vi "Initialize.vi"(8 "error in (no error)":errorcluster, 11 "Modbus master in":refnum<class "Modbus Master.lvclass">) -> (0 "error out":errorcluster, 3 "Modbus master out":refnum<class "Modbus Master.lvclass">)   [LabVIEW 2021, in "Modbus Master.lvclass"]
doc: "Initializes a Modbus master instance. If using the <B>Create Modbus Instance</B> VI, this is not necessary. This function will initiate any required bus communication."
uses:
  Modbus Master.lvclass
  D:/my_projects/projects/Algorithms/Labview/21/Modbus_v121c/API/Modbus API.lvclass
  Modbus API.lvclass/Modbus API.ctl
  Read Network Protocol.vi
  Network Protocol/Network Master/Network Master.lvclass
  D:/my_projects/projects/Algorithms/Labview/21/Modbus_v121c/Network Protocol/Network Protocol.lvclass
  Modbus API.lvclass
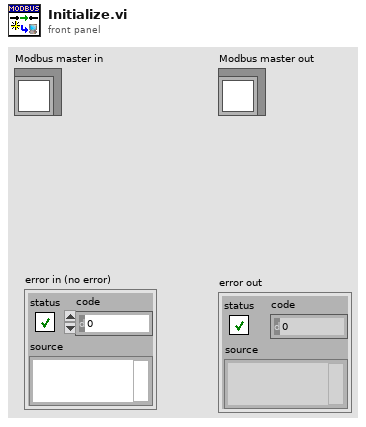
[diagram p1: front panel]
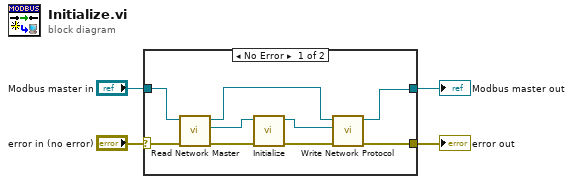
[diagram p0: block diagram]
diagram:
  n1 = case shown="No Error" "error in (no error)" {
    selector: "error in (no error)" -> [w12 w14]
    tunnel: [w7 w15] -> w4
    tunnel: "Modbus master in" -> [w11 w15]
    tunnel: [w8 w14] -> w2
    frame No Error {
      n2 = call "Read Network Master.vi"("error in"=w12, "Modbus master in"=w11) -> ("error out"=w5:errorcluster, "Network Master"=w6:refnum<class "Network Master.lvclass">, "Modbus master out"=w13:refnum<class "Modbus Master.lvclass">)  [unwired: 7 in]
      n3 = call-dynamic "Initialize.vi"("error in"=w5, "Network Master in"=w6) -> ("error out"=w9:errorcluster, "Network Master out"=w10:refnum<class "Network Master.lvclass">)  [unwired: 8 in]
      n4 = call "Write Network Protocol.vi"("error in (no error)"=w9, "Network Protocol"=w10, "Modbus API in"=w13) -> ("error out"=w8:errorcluster, "Modbus API out"=w7:refnum<class "Modbus Master.lvclass">)  [unwired: 7 in]
    }
    frame Error {
    }
  }
  "error out" <- w2
  "Modbus master out" <- w4
